vi "trimScreenshot.vi"(7 "Crop Rectangle":T2, 8 "error in (no error)":errorcluster, 11 "Flattened Image Data":T1) -> (0 "error out":errorcluster, 3 "Cropped Image Data":T1)   [LabVIEW 2018, in "Image_Diff.lvlib"]
uses:
  Image_Diff.lvlib
  <vilib>/picture/picture.llb/imagedata.ctl
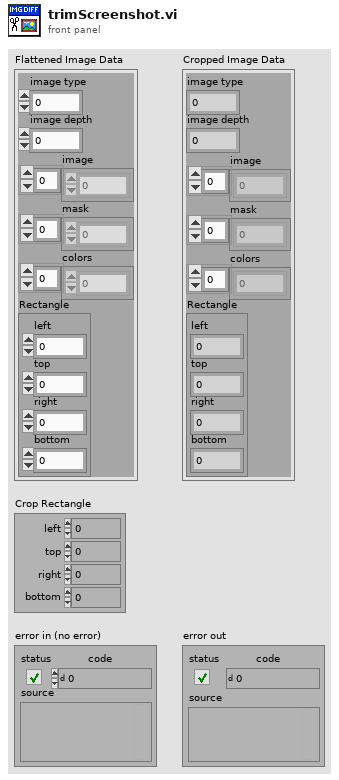
[diagram p1: front panel]
types:
  T1 = typedef "imagedata.ctl" = cluster{"image type":i32, "image depth":i32, "image":u8[], "mask":u8[], "colors":u32[], "Rectangle":cluster{"left":i16, "top":i16, "right":i16, "bottom":i16}}
  T2 = cluster{"left":i16, "top":i16, "right":i16, "bottom":i16}
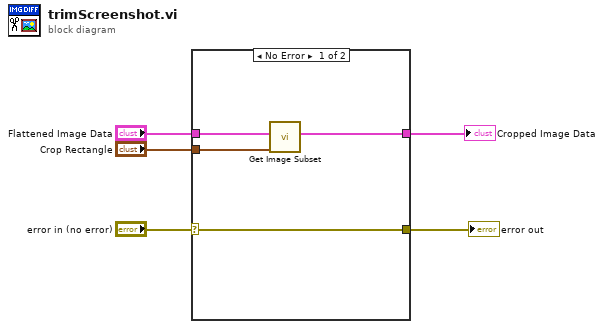
[diagram p0: block diagram]
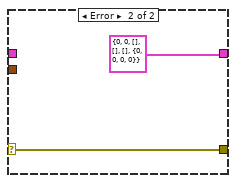
[diagram p2: hidden frame]
diagram:
  n1 = case shown="No Error" "error in (no error)" {
    selector: "error in (no error)" -> [w6 w10]
    tunnel: "Flattened Image Data" -> [w9 _]
    tunnel: "Crop Rectangle" -> [w8 _]
    tunnel: [w7 T1 {"image type"=0, "image depth"=0, "image"=[], "mask"=[], "colors"=[], "Rectangle"={"left"=0, "top"=0, "right"=0, "bottom"=0}} ("image subset")] -> w1
    tunnel: [w6 w10] -> w2
    frame No Error {
      n2 = call <vilib>:"Get Image Subset.vi"("subset rect"=w8, "image data"=w9) -> ("image subset"=w7:T1)  [unwired: 4 in, 1 out]
    }
    frame Error {
    }
  }
  "Cropped Image Data" <- w1
  "error out" <- w2
